vi "LifetimeCalculation.vi"(10 "S":dbl[][](array[numeric]), 11 "G":dbl[][](array[numeric])) -> (2 "DC&1w Lifetime":dbl[][](array[numeric]), 3 "1w Lifetime":dbl[][](array[numeric]))   [LabVIEW 2015]
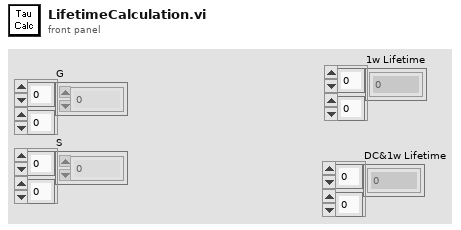
[diagram p1: front panel]
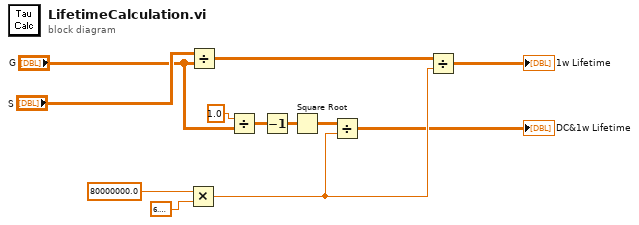
[diagram p0: block diagram]
diagram:
  n1 = Multiply(x=80000000.0, y=6.283185307179586) -> (x*y=w2:dbl)
  n2 = Divide(x="S", y="G") -> (x/y=w10:dbl[][])
  n3 = Divide(x=1.0, y="G") -> (x/y=w5:dbl[][])
  n4 = Decrement(x=w5) -> (x-1=w7:dbl[][])
  n5 = Square Root(x=w7) -> (sqrt(x)=w4:dbl[][])
  n6 = Divide(x=w4, y=w2) -> (x/y=→"DC&1w Lifetime":dbl[][])
  n7 = Divide(x=w10, y=w2) -> (x/y=→"1w Lifetime":dbl[][])
